vi "BRig_Host_comm_tcp_parseAccum_getCmd_first.vi"(10 "input_count":i32, 11 "input_strAccum":string) -> (0 "output_countCmd":i32, 1 "output_strCmd":string, 2 "output_count":i32, 3 "output_strAccum":string, 4 "output_I_cmd":bool)   [LabVIEW 2014]
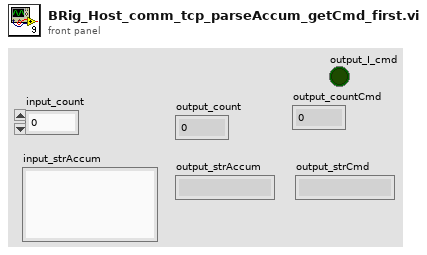
[diagram p1: front panel]
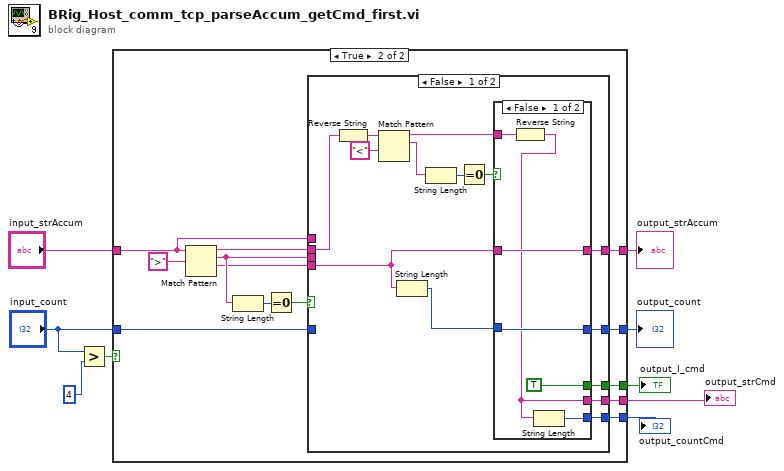
[diagram p0: block diagram]
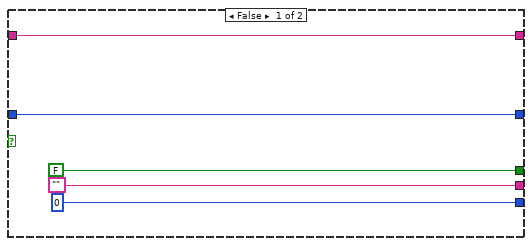
[diagram p2: hidden frame]
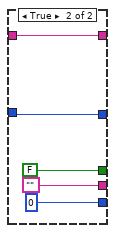
[diagram p3: hidden frame]
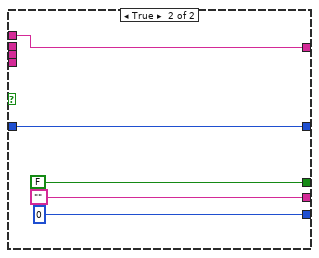
[diagram p4: hidden frame]
diagram:
  n1 = Greater?(x="input_count", y=4) -> (0:w7:bool)
  n2 = case shown="True" w7 {
    tunnel: "input_strAccum" -> [w10 w21]
    tunnel: [w10 w20] -> w5
    tunnel: "input_count" -> [w11 w19]
    tunnel: [w11 w18] -> w4
    tunnel: [FALSE w17] -> w3
    tunnel: ["" w16] -> w2
    tunnel: [u16 0 w15] -> w1
    frame False {
    }
    frame True {
      n3 = Match Pattern(string=w21, regular expression=">" ("search string/char (-)")) -> (before substring=w24:string, match substring=w23:string, after substring=w22:string)  [unwired: 1 in, 1 out]
      n4 = String Length(string=w23) -> (length=w26:i32)
      n5 = Equal To 0?(x=w26) -> (x = 0?=w25:bool)
      n6 = case shown="False" w25 {
        tunnel: w24 -> [w41 _]
        tunnel: w23 -> [_ _]
        tunnel: w22 -> [w29 _]
        tunnel: w21 -> [_ w57]
        tunnel: [w36 w57] -> w20
        tunnel: w19 -> [_ w56]
        tunnel: [w35 w56] -> w18
        tunnel: [w34 FALSE] -> w17
        tunnel: [w33 ""] -> w16
        tunnel: [w32 u16 0] -> w15
        frame False {
          n7 = Reverse String(1:w41) -> (0:w40:string)
          n8 = Match Pattern(string=w40, regular expression="<") -> (before substring=w31:string, match substring=w30:string)  [unwired: 1 in, 2 out]
          n9 = String Length(string=w29) -> (length=w28:i32)
          n10 = String Length(string=w30) -> (length=w38:i32)
          n11 = Equal To 0?(x=w38) -> (x = 0?=w37:bool)
          n12 = case shown="False" w37 {
            tunnel: [w47 w48] -> w36
            tunnel: [w46 w49] -> w35
            tunnel: [TRUE FALSE] -> w34
            tunnel: [w42 ""] -> w33
            tunnel: [w44 u16 0] -> w32
            tunnel: w31 -> [w43 _]
            tunnel: w28 -> [w46 w49]
            tunnel: w29 -> [w47 w48]
            frame False {
              n13 = Reverse String(1:w43) -> (0:w42:string)
              n14 = String Length(string=w42) -> (length=w44:i32)
            }
            frame True {
            }
          }
        }
        frame True {
        }
      }
    }
  }
  "output_strAccum" <- w5
  "output_count" <- w4
  "output_I_cmd" <- w3
  "output_strCmd" <- w2
  "output_countCmd" <- w1
